vi "Simulate Keysight 34401a TCP.vi"() -> ()   [LabVIEW 2020, in "Keysight_34401A-DMM.lvclass"]
uses:
  Keysight_34401A-DMM.lvclass
  <vilib>/Utility/config.llb/Read Key (String).vi
  <vilib>/Utility/config.llb/NI_LVConfig.lvlib
panel:
  out "error out":errorcluster
  in  "stop":bool
  in  "timeout ms (wait forever: -1)":i32=1000
  in  "port":u16=50000
  in  "error in":errorcluster
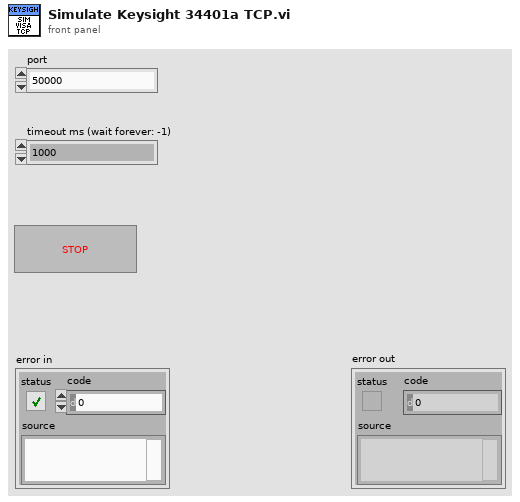
[diagram p1: front panel]
types:
  T1 = typedef "NI_LVConfig.lvlib/Config Data RefNum.ctl" = refnum<k1>
  T2 = enum16{"Standard", "Buffered", "CRLF", "Immediate"}
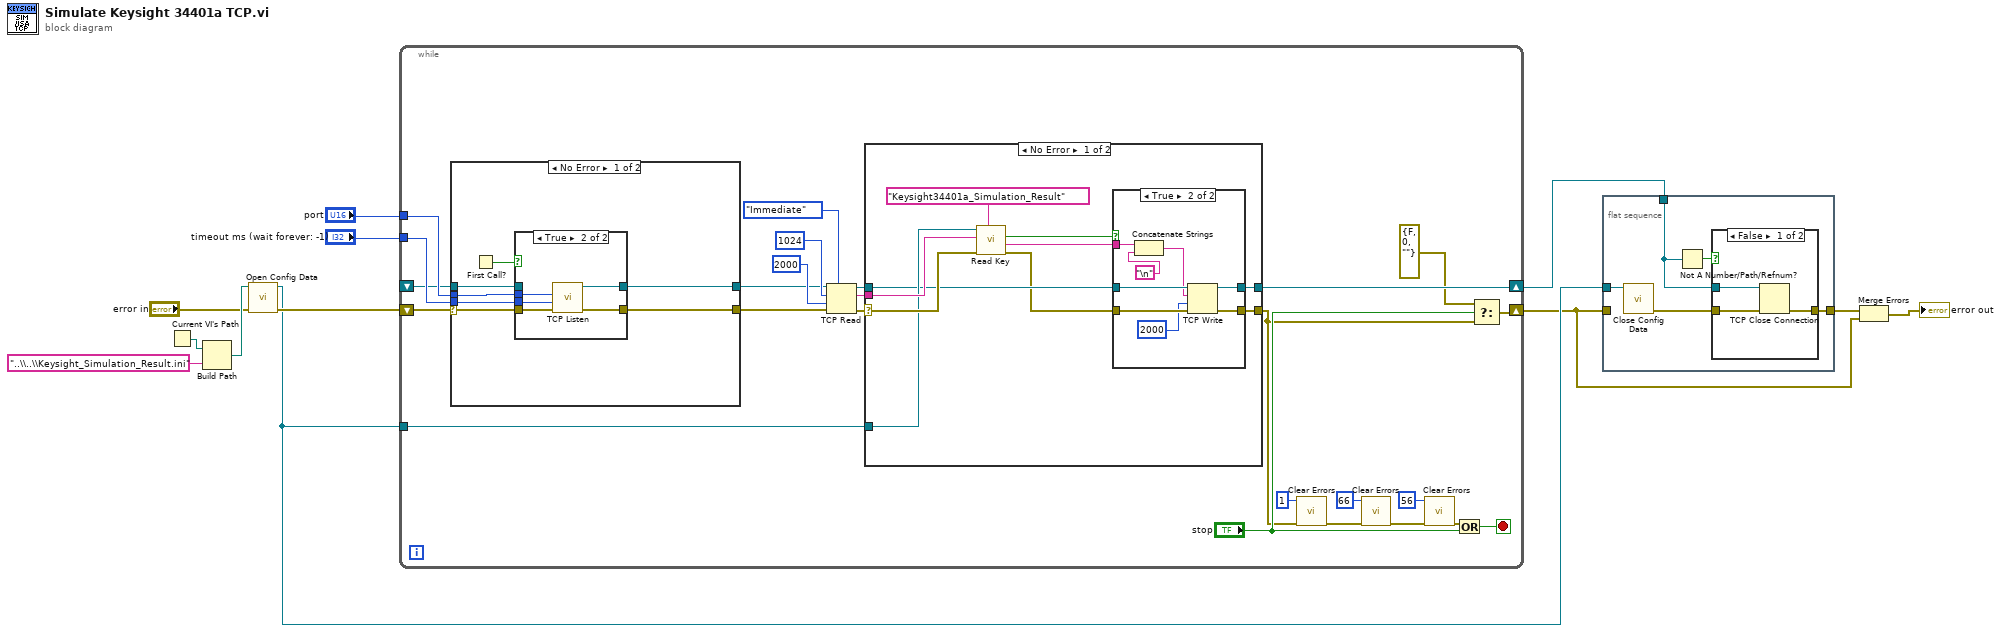
[diagram p0: block diagram]
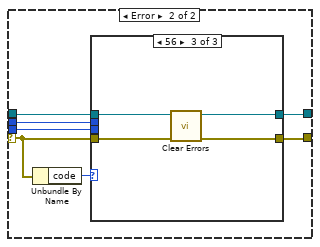
[diagram p5: hidden frame]
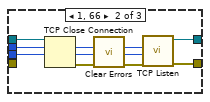
[diagram p7: hidden frame]
diagram:
  n1 = Current VI's Path() -> (path=w12:path)
  n2 = Build Path(base path=w12, name or relative path="..\\..\\Keysight_Simulation_Result.ini" ("write buffer")) -> (appended path=w10:path)
  n3 = call <vilib>:"Open Config Data.vi"("error in (no error)"="error in", "configuration file path"=w10) -> ("error out"=w8:errorcluster, "refnum"=w7:T1)  [unwired: 7 in, 1 out]
  n4 = while {
    tunnel: w7 -> [w32]
    tunnel: "port" -> [w25]
    tunnel: "timeout ms (wait forever: -1)" -> [w24]
    shift-right: [w13] -> w4
    shift-left: w8 -> [w26]
    shift-right: [w28] -> w3
    shift-left: _ -> [w19]
    stop <- w30 stop-if-true
    n5 = case shown="No Error" w26 {
      selector: w26 -> [w64 w78]
      tunnel: [w66 w77] -> w29
      tunnel: [w65 w79] -> w27
      tunnel: w25 -> [w63 w76]
      tunnel: w24 -> [w62 w75]
      tunnel: w19 -> [w60 w74]
      frame No Error {
        n6 = First Call?() -> (First Call?: T/F=w61:bool)
        n7 = case shown="True" w61 {
          tunnel: [w67 w73] -> w66
          tunnel: [w68 w72] -> w65
          tunnel: w64 -> [w68 w71]
          tunnel: w63 -> [_ w70]
          tunnel: w62 -> [_ w69]
          tunnel: w60 -> [w67 _]
          frame False {
          }
          frame True {
            n8 = call <vilib>:"TCP Listen.vi"("error in (no error)"=w71, "timeout ms (wait forever: -1)"=w69, "port"=w70) -> ("error out"=w72:errorcluster, "connection ID"=w73:refnum<k5>)  [unwired: 4 in, 3 out]
          }
        }
      }
      frame Error {
        n9 = Unbundle By Name(w78) -> ("code"=w80:i32)
        n10 = case shown="56" w80 {
          tunnel: [w82 w89 w90] -> w79
          tunnel: w78 -> [w82 _ w92]
          tunnel: [w81 w88 w91] -> w77
          tunnel: w76 -> [_ w87 _]
          tunnel: w75 -> [_ w86 _]
          tunnel: w74 -> [w81 w84 w91]
          frame Default {
          }
          frame 1, 66 {
            n11 = TCP Close Connection(connection ID=w84) -> (error out=w85:errorcluster)  [unwired: 2 in, 1 out]
            n12 = call <vilib>:"Clear Errors.vi"("error in (no error)"=w85) -> ("error out"=w83:errorcluster)  [unwired: 5 in, 1 out]
            n13 = call <vilib>:"TCP Listen.vi"("error in (no error)"=w83, "timeout ms (wait forever: -1)"=w86, "port"=w87) -> ("error out"=w89:errorcluster, "connection ID"=w88:refnum<k5>)  [unwired: 4 in, 3 out]
          }
          frame 56 {
            n14 = call <vilib>:"Clear Errors.vi"("error in (no error)"=w92) -> ("error out"=w90:errorcluster)  [unwired: 5 in, 1 out]
          }
        }
      }
    }
    n15 = TCP Read(connection ID=w29, bytes to read=1024, error in (no error)=w27, 7:T2."Immediate" ("mode (standard)"), 9:2000 ("timeout ms (25000)")) -> (connection ID out=w31:refnum<k5>, data out=w33:string, error out=w34:errorcluster)
    n16 = case shown="No Error" w34 {
      selector: w34 -> [w47 w58]
      tunnel: w33 -> [w46 _]
      tunnel: w32 -> [w45 _]
      tunnel: w31 -> [w44 w59]
      tunnel: [w43 w58] -> w15
      tunnel: [w42 w59] -> w28
      frame No Error {
        n17 = call-poly <vilib>:"Read Key.vi"("section"="Keysight34401a_Simulation_Result", "error in (no error)"=w47, "key"=w46, "refnum"=w45) -> ("error out"=w40:errorcluster, "value"=w39:string, "found?"=w38:bool)  [unwired: 4 in, 1 out]
        n18 = case shown="True" w38 {
          tunnel: w40 -> [w49 w57]
          tunnel: [w49 w56] -> w43
          tunnel: w44 -> [w48 w55]
          tunnel: w39 -> [_ w53]
          tunnel: [w48 w52] -> w42
          frame False {
          }
          frame True {
            n19 = Concatenate Strings(w53, "\n") -> (w51:string)
            n20 = TCP Write(connection ID=w55, data in=w51, error in (no error)=w57, 9:2000 ("timeout ms (25000)")) -> (connection ID out=w52:refnum<k5>, error out=w56:errorcluster)  [unwired: 1 out]
          }
        }
      }
      frame Error {
      }
    }
    n21 = call <vilib>:"Clear Errors.vi"("error in (no error)"=w15, "specific error code to clear (0: all)"=1) -> ("error out"=w18:errorcluster)  [unwired: 4 in, 1 out]
    n22 = call <vilib>:"Clear Errors.vi"("error in (no error)"=w18, "specific error code to clear (0: all)"=66) -> ("error out"=w21:errorcluster)  [unwired: 4 in, 1 out]
    n23 = call <vilib>:"Clear Errors.vi"("error in (no error)"=w21, "specific error code to clear (0: all)"=56) -> ("error out"=w23:errorcluster)  [unwired: 4 in, 1 out]
    n24 = Or(x=w23, y="stop") -> (x .or. y?=w30:bool)
    n25 = Select(t=errorcluster {"status"=FALSE, "code"=0, "source"=""}, s="stop", f=w15) -> (s? t:f=w13:errorcluster)
  }
  n26 = flat-sequence {
    tunnel: w7 -> [w97]
    tunnel: [w95] -> w6
    tunnel: w3 -> [w94]
    tunnel: w4 -> [_]
    frame #0 {
      n27 = call <vilib>:"Close Config Data.vi"("refnum"=w97) -> ("error out"=w96:errorcluster)  [unwired: 9 in, 1 out]
      n28 = Not A Number/Path/Refnum?(number/path/refnum=w94) -> (NaN/Path/Refnum?=w93:bool)
      n29 = case shown="False" w93 {
        tunnel: w96 -> [w100 w101]
        tunnel: [w99 w101] -> w95
        tunnel: w94 -> [w98 _]
        frame False {
          n30 = TCP Close Connection(connection ID=w98, error in (no error)=w100) -> (error out=w99:errorcluster)  [unwired: 1 in, 1 out]
        }
        frame True {
        }
      }
    }
  }
  n31 = Merge Errors(w6, w4) -> (→"error out":errorcluster)
